vi "ProdaNG.Tree.Add.vi"(5 "Identification":T1, 6 "reason":string, 7 "TestStepsTree":refnum<vi>, 8 "error in (no error)":errorcluster, 9 "Element values":T2, 10 "Element to add":T3, 11 "dbHandleIn":i32) -> (0 "error out":errorcluster, 3 "dbHandle":i32)   [LabVIEW 2016]
uses:
  ProdaNG.Tree.Fglb.Data.ctl
  ProdaNG.Tree.Fglb.Element.ctl
  ProdaNG.Tree.Fglb.Value.ctl
  Controls/ProdaNG.ProcessStepParam.ctl
  Controls/ProdaNG.TestStep.ctl
  Controls/ProdaNG.TestStepParam.ctl
  Controls/ProdaNG.TestValue.ctl
  ProdaNG.Configurator.Glb.vi
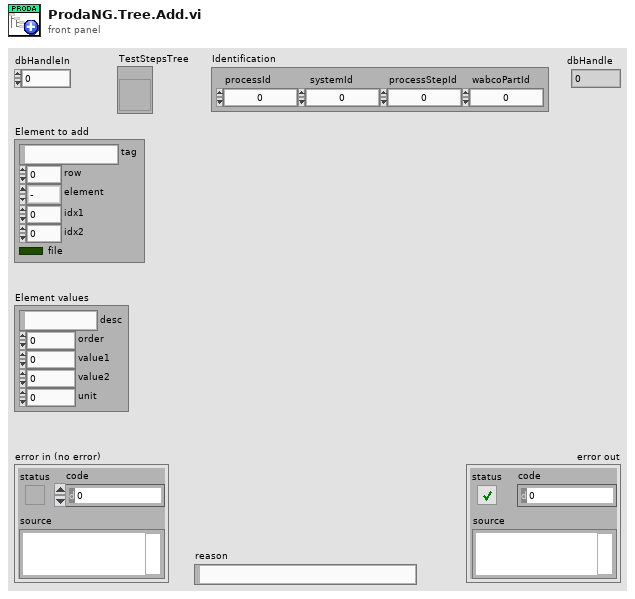
[diagram p1: front panel]
types:
  T1 = cluster{"processId":i32, "systemId":i32, "processStepId":i32, "wabcoPartId":i32}
  T2 = typedef "ProdaNG.Tree.Fglb.Value.ctl" = cluster{"desc":string, "order":i32, "value1":dbl, "value2":dbl, "unit":i32}
  T3 = typedef "ProdaNG.Tree.Fglb.Data.ctl" = cluster{"tag":string, "row":i32, "element":T4, "idx1":i32, "idx2":i32, "file":bool}
  T4 = typedef "ProdaNG.Tree.Fglb.Element.ctl" = enum16{"-", "PP", "TS", "TP", "TV"}
  T5 = typedef "ProdaNG.ProcessStepParam.ctl" = cluster{"i_id":i32, "processStepId":i32, "unitId":i32, "contentId":string, "previewId":string, "value":dbl, "valueText":string, "paramSequence":i32, "history":i32, "mdReason":string, "mdUser":string, "mdTime":string, "description":string}
  T6 = typedef "ProdaNG.TestStep.ctl" = cluster{"i_id":i32, "processStepId":i32, "testSequence":i32, "testOrder":i32, "mdReason":string, "mdUser":string, "mdTime":string, "description":string}
  T7 = typedef "ProdaNG.TestStepParam.ctl" = cluster{"i_id":i32, "testStepId":i32, "unitId":i32, "contentId":string, "previewId":string, "value":dbl, "valueText":string, "paramSequence":i32, "history":i32, "mdReason":string, "mdUser":string, "mdTime":string, "description":string}
  T8 = typedef "ProdaNG.TestValue.ctl" = cluster{"i_id":i32, "testStepId":i32, "releaseId":i32, "unitId":i32, "contentId":string, "previewId":string, "maximum":dbl, "minimum":dbl, "valueText":string, "testValueSequence":i32, "history":i32, "mdReason":string, "mdUser":string, "mdTime":string, "description":string}
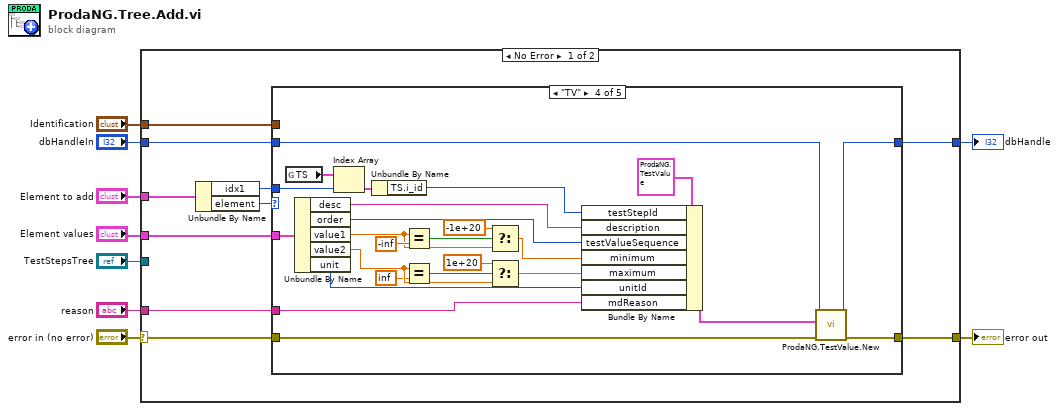
[diagram p0: block diagram]
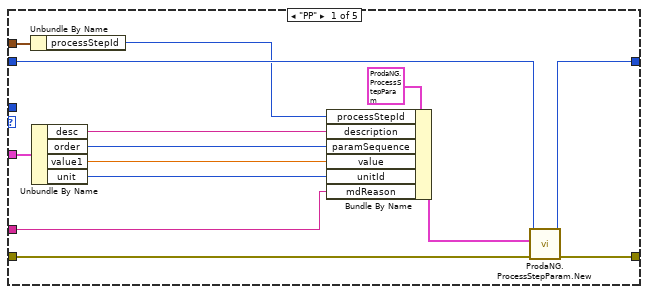
[diagram p2: hidden frame]
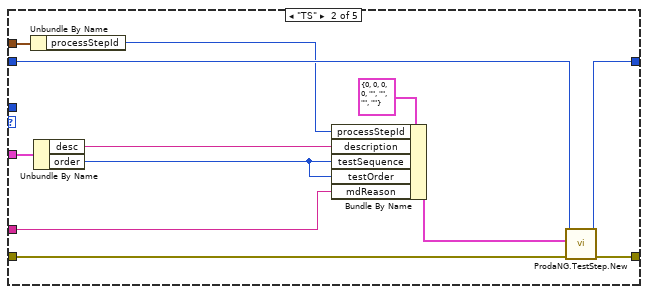
[diagram p3: hidden frame]
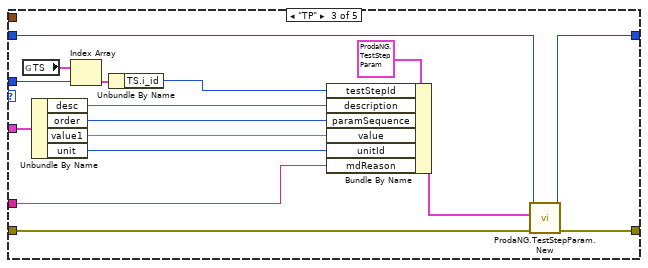
[diagram p4: hidden frame]
diagram:
  n1 = case shown="No Error" "error in (no error)" {
    selector: "error in (no error)" -> [w15 w90]
    tunnel: "TestStepsTree" -> [_ _]
    tunnel: [w19 w90] -> w9
    tunnel: "dbHandleIn" -> [w18 w89]
    tunnel: [w17 w89] -> w5
    tunnel: "Element to add" -> [w16 _]
    tunnel: "Element values" -> [w14 _]
    tunnel: "reason" -> [w13 _]
    tunnel: "Identification" -> [w12 _]
    frame No Error {
      n2 = Unbundle By Name(w16) -> ("idx1"=w10:i32, "element"=w11:T4)
      n3 = case shown="\"TV\"" w11 {
        tunnel: w15 -> [w30 w45 w57 w83 w88]
        tunnel: [w33 w44 w60 w86 w88] -> w19
        tunnel: w18 -> [w32 w43 w59 w85 w87]
        tunnel: [w31 w42 w58 w84 w87] -> w17
        tunnel: w14 -> [w29 w40 w56 w82 _]
        tunnel: w13 -> [w24 w35 w49 w76 _]
        tunnel: w12 -> [w22 w38 _ _ _]
        tunnel: w10 -> [_ _ w50 w67 _]
        frame "PP" {
          n4 = Unbundle By Name(w22) -> ("processStepId"=w21:i32)
          n5 = Unbundle By Name(w29) -> ("desc"=w28:string, "order"=w27:i32, "value1"=w26:dbl, "unit"=w20:i32)
          n6 = Bundle By Name(cluster=T5 {"i_id"=0, "processStepId"=0, "unitId"=0, "contentId"="", "previewId"="", "value"=0.0, "valueText"="", "paramSequence"=0, "history"=0, "mdReason"="", "mdUser"="", "mdTime"="", "description"=""} ("element"), "processStepId"=w21, "description"=w28, "paramSequence"=w27, "value"=w26, "unitId"=w20, "mdReason"=w24) -> (w25:T5)
          n7 = call "ProdaNG.ProcessStepParam.New.vi"("error in (no error)"=w30, "ProcessStepParam"=w25, "dbHandleIn"=w32) -> ("error out"=w33:errorcluster, "dbHandle"=w31:i32)  [unwired: 6 in, 1 out]
        }
        frame "TS" {
          n8 = Unbundle By Name(w38) -> ("processStepId"=w36:i32)
          n9 = Unbundle By Name(w40) -> ("desc"=w41:string, "order"=w34:i32)
          n10 = Bundle By Name(cluster=T6 {"i_id"=0, "processStepId"=0, "testSequence"=0, "testOrder"=0, "mdReason"="", "mdUser"="", "mdTime"="", "description"=""} ("TestStep"), "processStepId"=w36, "description"=w41, "testSequence"=w34, "testOrder"=w34, "mdReason"=w35) -> (w39:T6)
          n11 = call "ProdaNG.TestStep.New.vi"("error in (no error)"=w45, "TestStep"=w39, "dbHandleIn"=w43) -> ("error out"=w44:errorcluster, "dbHandle"=w42:i32)  [unwired: 6 in, 1 out]
        }
        frame "TP" {
          n12 = global read "ProdaNG.Configurator.Glb.vi" "TS"() -> (w61:cluster{"TS":T6, "TP":T7[], "TV":T8[]}[])
          n13 = Unbundle By Name(w56) -> ("desc"=w55:string, "order"=w54:i32, "value1"=w53:dbl, "unit"=w47:i32)
          n14 = Index Array(array=w61, index=w50) -> (element=w51:cluster{"TS":T6, "TP":T7[], "TV":T8[]})
          n15 = Unbundle By Name(w51) -> ("TS.i_id"=w46:i32)
          n16 = Bundle By Name(cluster=T7 {"i_id"=0, "testStepId"=0, "unitId"=0, "contentId"="", "previewId"="", "value"=0.0, "valueText"="", "paramSequence"=0, "history"=0, "mdReason"="", "mdUser"="", "mdTime"="", "description"=""} ("TestStepParam"), "testStepId"=w46, "description"=w55, "paramSequence"=w54, "value"=w53, "unitId"=w47, "mdReason"=w49) -> (w52:T7)
          n17 = call "ProdaNG.TestStepParam.New.vi"("error in (no error)"=w57, "TestStepParam"=w52, "dbHandleIn"=w59) -> ("error out"=w60:errorcluster, "dbHandle"=w58:i32)  [unwired: 6 in, 1 out]
        }
        frame "TV" {
          n18 = global read "ProdaNG.Configurator.Glb.vi" "TS"() -> (w69:cluster{"TS":T6, "TP":T7[], "TV":T8[]}[])
          n19 = Unbundle By Name(w82) -> ("desc"=w64:string, "order"=w65:i32, "value1"=w79:dbl, "value2"=w72:dbl, "unit"=w62:i32)
          n20 = Index Array(array=w69, index=w67) -> (element=w68:cluster{"TS":T6, "TP":T7[], "TV":T8[]})
          n21 = Unbundle By Name(w68) -> ("TS.i_id"=w63:i32)
          n22 = Equal?(x=w79, y=-inf) -> (x = y?=w78:bool)
          n23 = Equal?(x=w72, y=inf) -> (x = y?=w73:bool)
          n24 = Select(t=-1e+20, s=w78, f=w79) -> (s? t:f=w75:dbl)
          n25 = Select(t=1e+20, s=w73, f=w72) -> (s? t:f=w70:dbl)
          n26 = Bundle By Name(cluster=T8 {"i_id"=0, "testStepId"=0, "releaseId"=0, "unitId"=0, "contentId"="", "previewId"="", "maximum"=0.0, "minimum"=0.0, "valueText"="", "testValueSequence"=0, "history"=0, "mdReason"="", "mdUser"="", "mdTime"="", "description"=""} ("TestValue"), "testStepId"=w63, "description"=w64, "testValueSequence"=w65, "minimum"=w75, "maximum"=w70, "unitId"=w62, "mdReason"=w76) -> (w81:T8)
          n27 = call "ProdaNG.TestValue.New.vi"("error in (no error)"=w83, "TestValue"=w81, "dbHandleIn"=w85) -> ("error out"=w86:errorcluster, "dbHandle"=w84:i32)  [unwired: 6 in, 1 out]
        }
        frame Default {
        }
      }
    }
    frame Error {
    }
  }
  "error out" <- w9
  "dbHandle" <- w5
